vi "TestFunction.vi"() -> ()   [LabVIEW 2023]
panel:
  out "error out":errorcluster
  out "session out":refnum<k37>
  in  "error in (no error)":errorcluster
  in  "source file path":path
  out "op":dbl
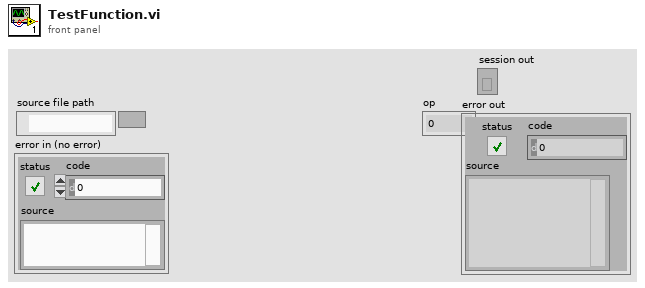
[diagram p1: front panel]
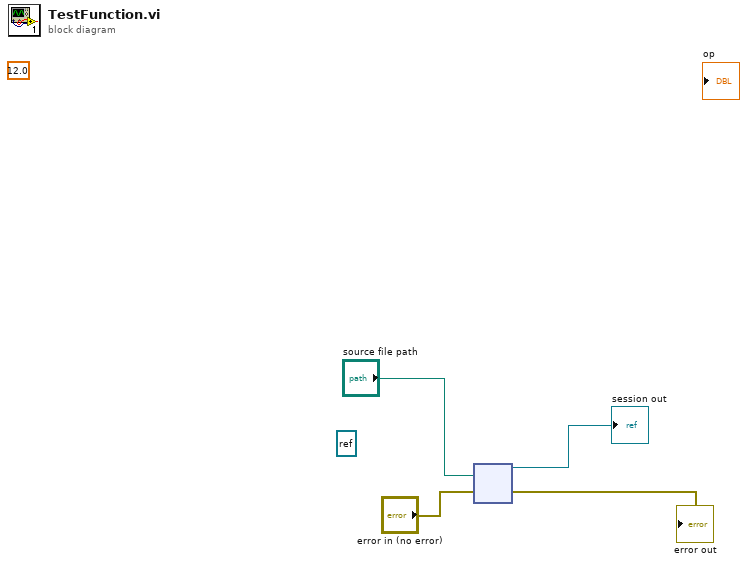
[diagram p0: block diagram]
diagram:
  (unwired) refnum<k37> refnum ("session in")
  (unwired) 12.0 ("Real")
  n1 = node("source file path", "error in (no error)") -> (w5:refnum<k37>, →"session out":refnum<k37>, →"error out":errorcluster)  [unwired: 3 in, 2 out]
